vi "Global_CMD_Gear.vi"() -> ()   [LabVIEW 2016]
panel:
  in  "CMD_Gear_High(T)Low(F)":bool
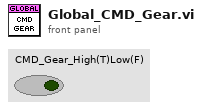
[diagram p1: front panel]
diagram:
